vi "Show_results_files.vi"() -> ()   [LabVIEW 2010]
panel:
  out "List of Filenames":path[](array[path])
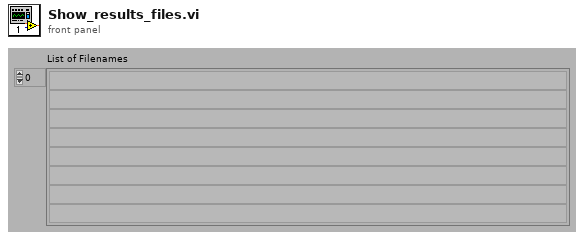
[diagram p1: front panel]
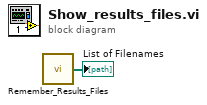
[diagram p0: block diagram]
diagram:
  n1 = call "Remember_Results_Files.vi"() -> ("List of Filenames"=→"List of Filenames":path[])  [unwired: 1 in]
